vi "State Change.vi"(8 "error in":errorcluster, 10 "Transition State":refnum<class "State Pattern.lvclass">, 11 "Context in":refnum<class "State Pattern.lvclass">) -> (0 "error out":errorcluster, 3 "Context out":refnum<class "State Pattern.lvclass">)   [LabVIEW 2021, in "State Pattern.lvclass"]
uses:
  State Pattern.lvclass
panel:
  # "This IS the same object coming out, so is at the top right instead of on the connector terminal below"
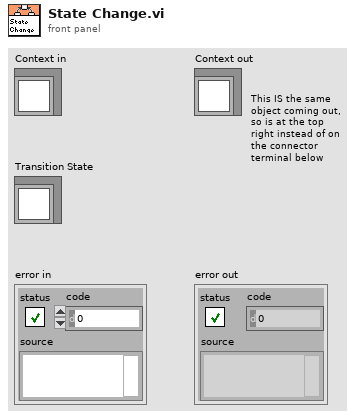
[diagram p1: front panel]
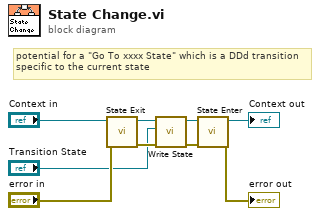
[diagram p0: block diagram]
diagram:
  # "potential for a \"Go To xxxx State\" which is a DDd transition specific to the current state"
  n1 = call "State Exit.vi"("error in"="error in", "Context in"="Context in") -> ("error out"=w9:errorcluster, "Context out"=w5:refnum<class "State Pattern.lvclass">)  [unwired: 8 in]
  n2 = call-dynamic "Write State.vi"("error in"=w9, "State"="Transition State", "Context in"=w5) -> ("error out"=w8:errorcluster, "Context out"=w4:refnum<class "State Pattern.lvclass">)  [unwired: 7 in]
  n3 = call "State Enter.vi"("error in"=w8, "Context in"=w4) -> ("error out"=→"error out":errorcluster, "Context out"=→"Context out":refnum<class "State Pattern.lvclass">)  [unwired: 8 in]
